vi "playlist_test.vi"() -> ()   [LabVIEW 2010]
uses:
  System.Windows.Forms
  <vilib>/Utility/miscctls.llb/LVPoint32TypeDef.ctl
  <vilib>/Utility/error.llb/DialogType.ctl
  musicplayer_glo.vi
  <vilib>/Utility/inputDevices.llb/mouseAcquire.vi
  shell32.dll
  user32.dll
panel:
  out "file count":u32
  out "drop-array":string[](array[string])
  out "win msg queue":T1
  in  "cancel":bool
  in  "ProgressBar":refnum<k24>(container)
  out "verdeckung":bool=TRUE
  in  "playlist":i32[](listbox)=[-2] caption="Playlist"
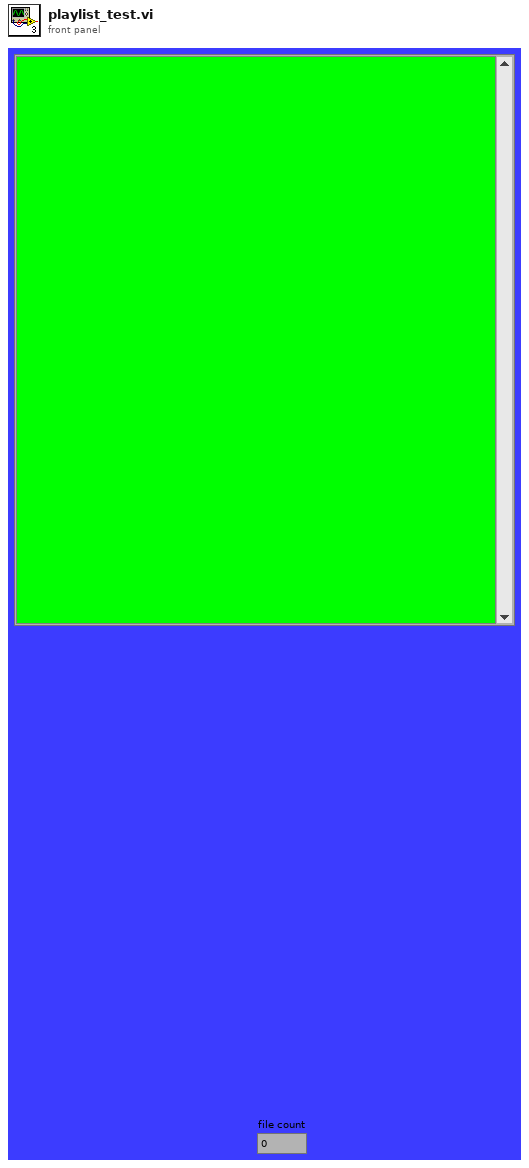
[diagram p1: front panel]
types:
  T1 = typedef "Win Msg Queue RefNum" = refnum<k1>
  T2 = enum8{"Enabled", "Disabled", "Disabled and Grayed Out"}
  T3 = enum32{"Invalid", "Standard", "Closed", "Hidden", "Minimized", "Maximized"}
  T4 = typedef "LVPoint32TypeDef.ctl" = cluster{"Horizontal":i32, "Vertical":i32}
  T5 = enum32{"Invalid", "Default", "Floating", "Floating/Auto-Hide", "Modal"}
  T6 = cluster{"Horizontal":i32, "Vertical":i32, "Scrolling":i32}
  T7 = cluster{"hWnd":u32, "Msg":u32, "wParam":u32, "lParam":i32, "time":u32, "point":cluster{"X":i32, "Y":i32}}
  T8 = typedef "DialogType.ctl" = u16
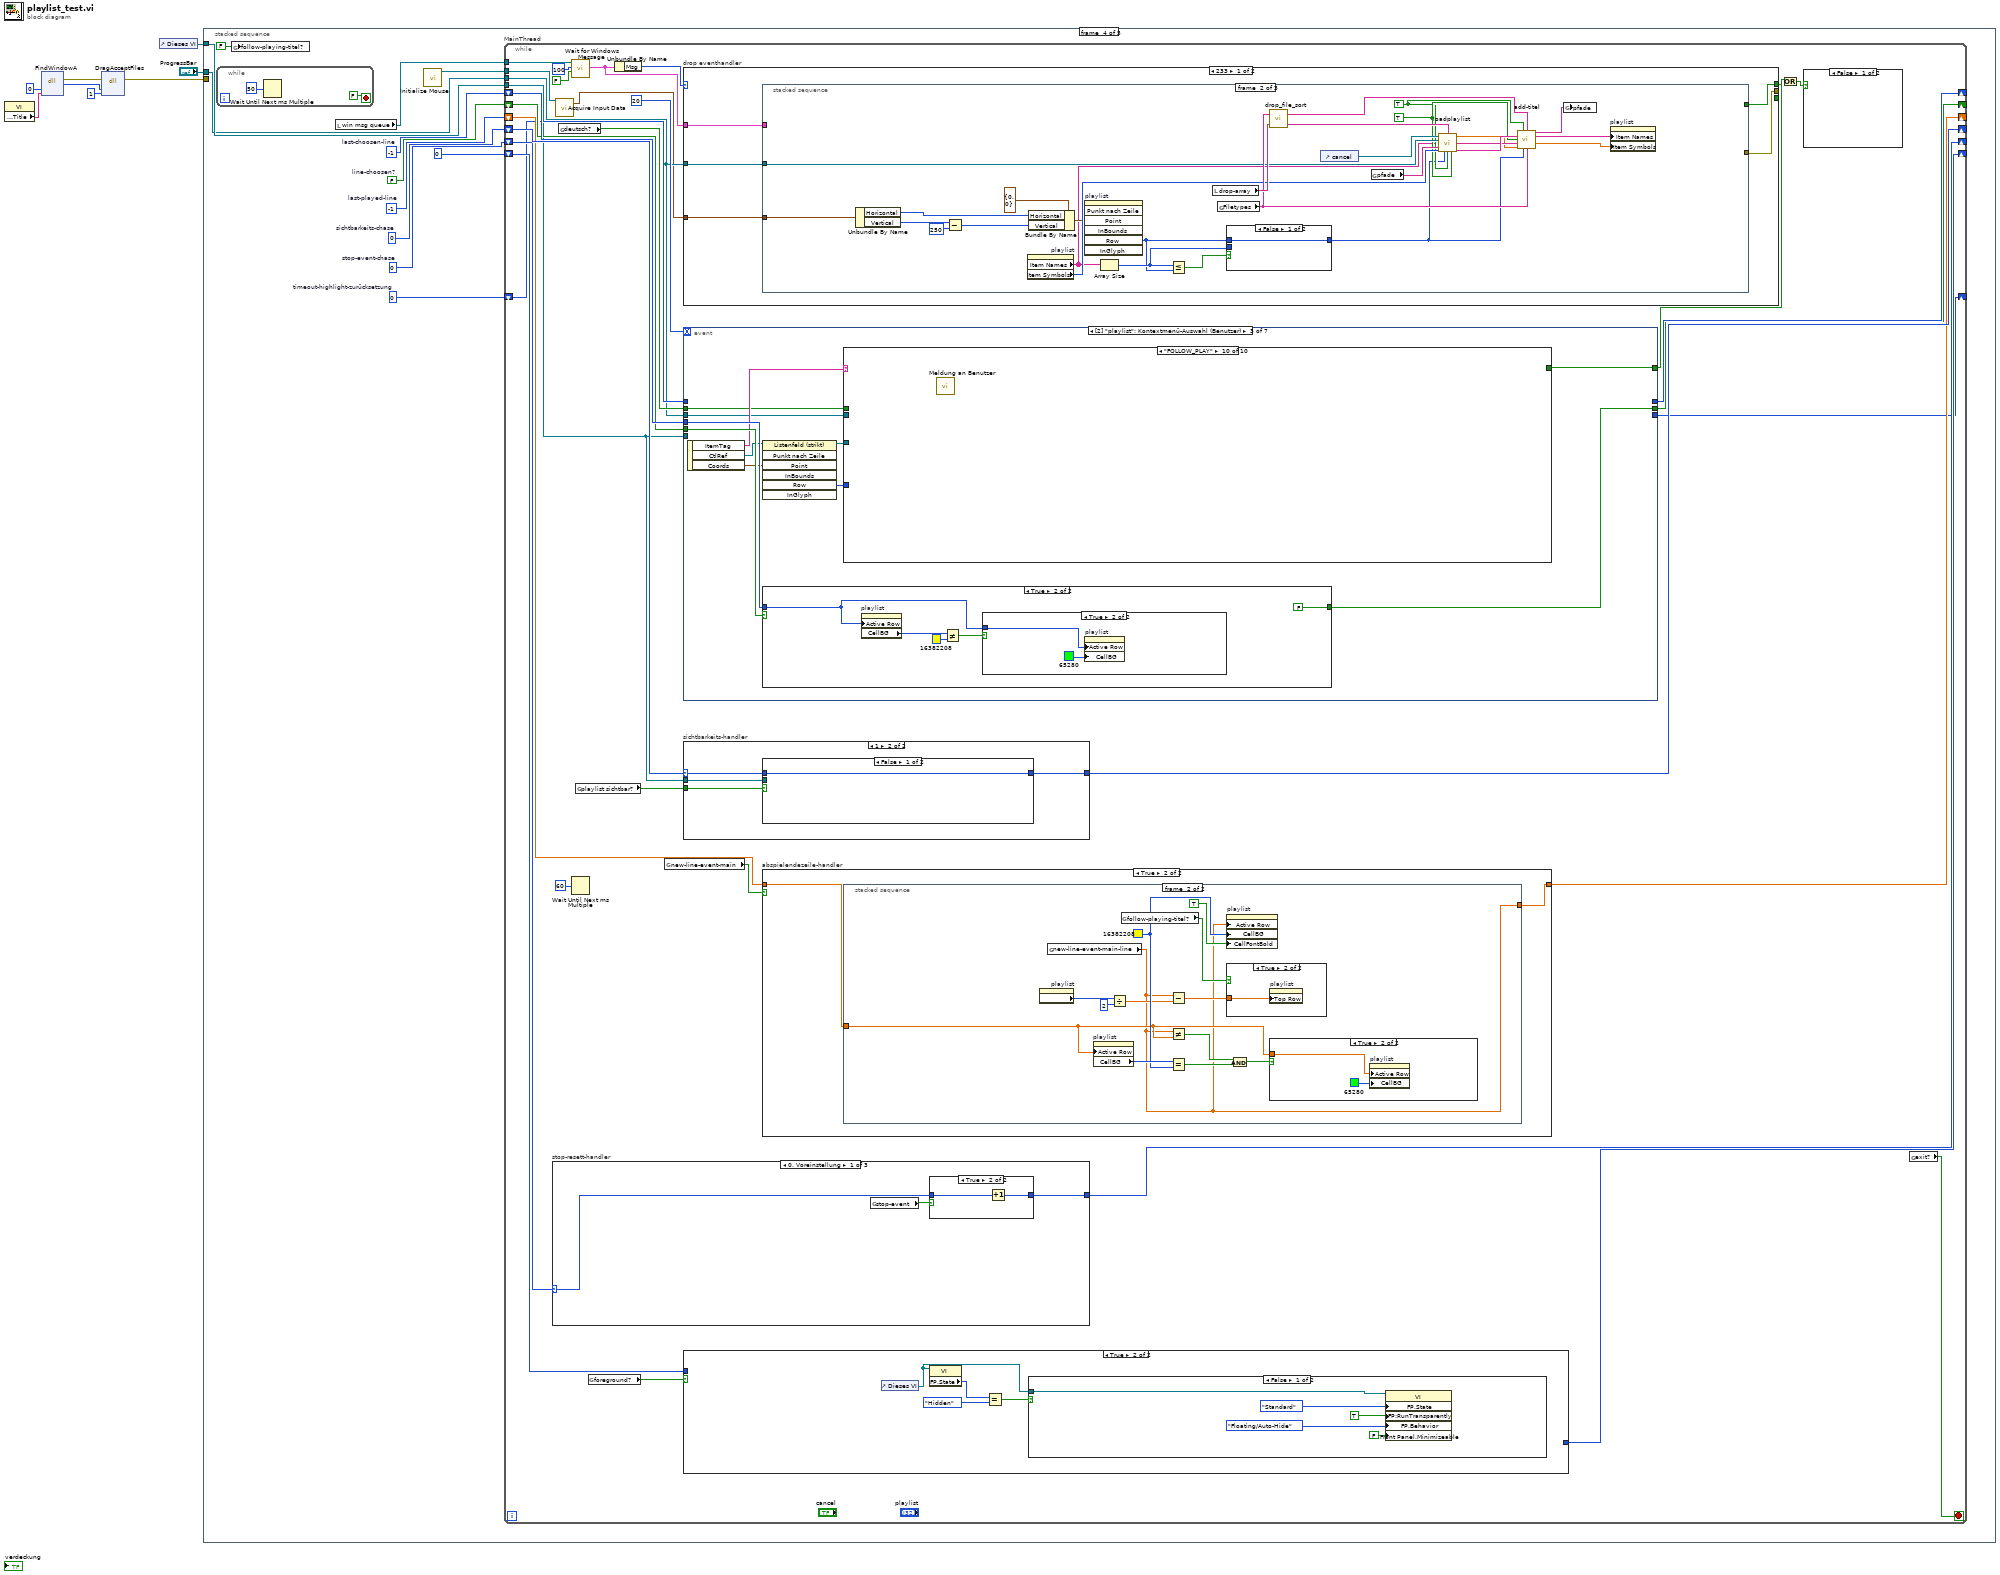
[diagram p0: block diagram]
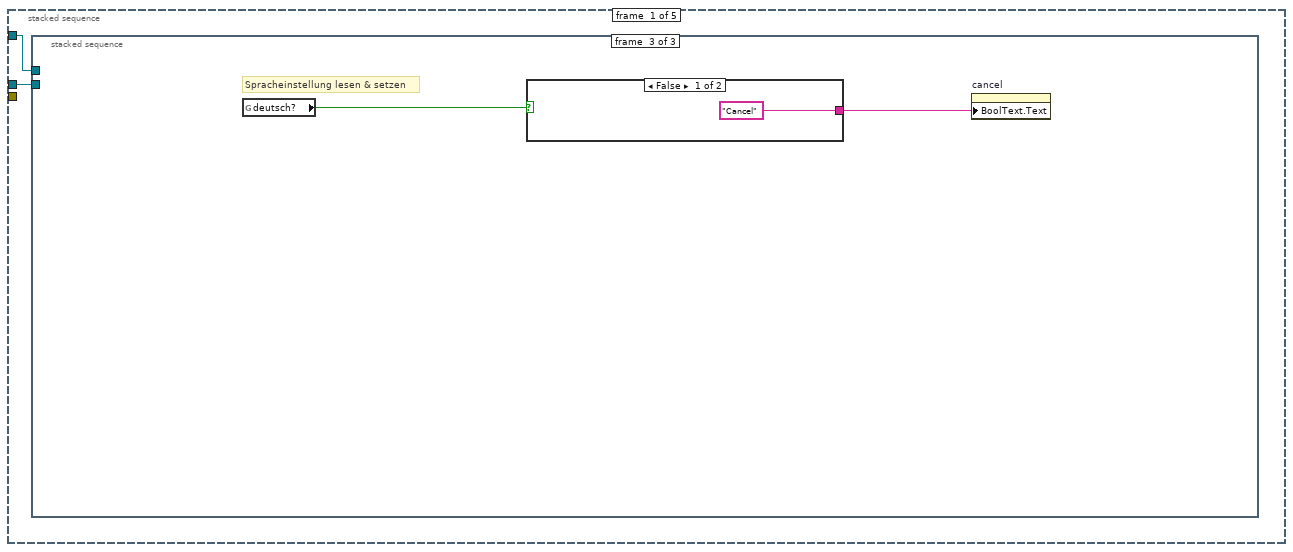
[diagram p2: hidden frame]
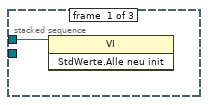
[diagram p3: hidden frame]
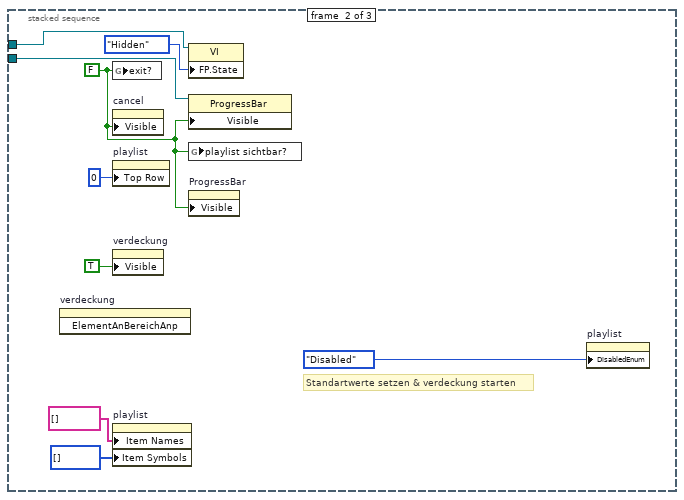
[diagram p4: hidden frame]
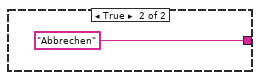
[diagram p5: hidden frame]
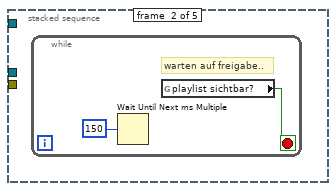
[diagram p6: hidden frame]
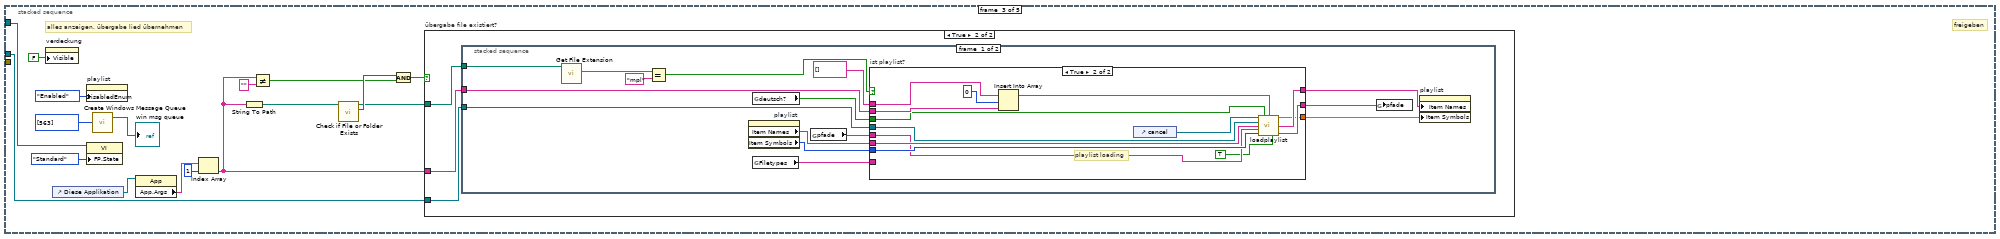
[diagram p7: hidden frame]
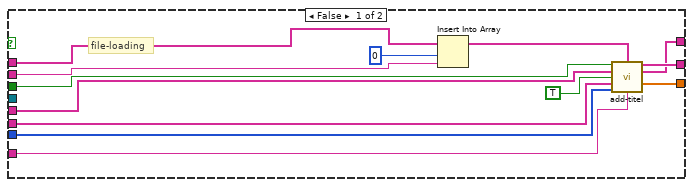
[diagram p9: hidden frame]
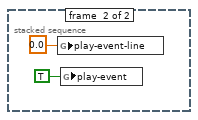
[diagram p10: hidden frame]
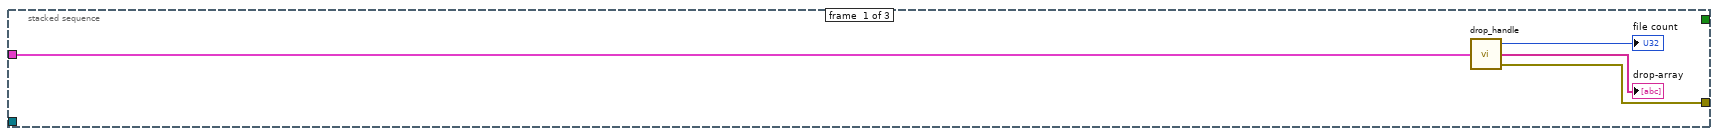
[diagram p11: hidden frame]
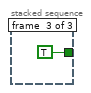
[diagram p13: hidden frame]
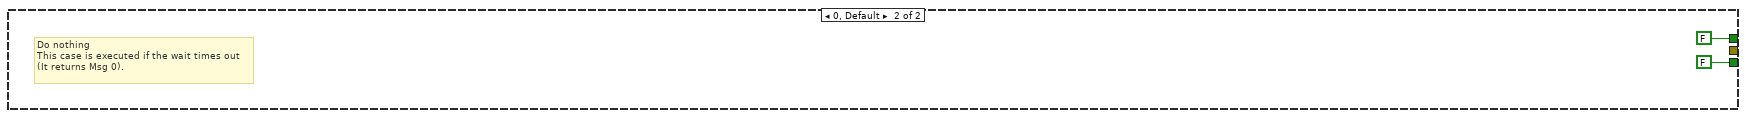
[diagram p14: hidden frame]
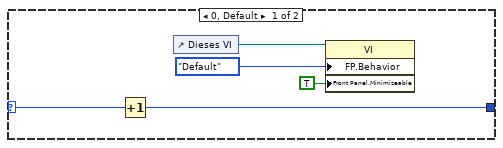
[diagram p16: hidden frame]
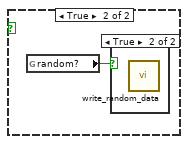
[diagram p18: hidden frame]
diagram:
  n1 = property class="VI"() -> ("Front Panel Window:Title"=w5:string)  [unwired: 2 in, 2 out]
  n2 = dll-call lib="user32.dll" fn="FindWindowA" label="FindWindow"("lpszClassName"=0, "lpszWindowName"=w5) -> (error out=w6:errorcluster, "hWnd"=w2:u32)  [unwired: 5 in, 1 out]
  n3 = dll-call lib="shell32.dll" fn="DragAcceptFiles"(error in=w6, "hWnd"=w2, "fAccept"=1) -> (error out=w1:errorcluster)  [unwired: 5 in, 1 out]
  n4 = control-ref of="Dieses VI"() -> (w8:refnum<vi>)
  n5 = stacked-sequence {
    tunnel: w8 -> [w10 _ w41 w102 w420]
    tunnel: "ProgressBar" -> [w9 _ w27 w97 _]
    tunnel: w1 -> [_ _ _ _ _]
    frame #0 {
      n6 = stacked-sequence {
        tunnel: w10 -> [w11 w17 _]
        tunnel: w9 -> [_ w13 _]
        frame #0 {
          n7 = invoke class="VI" method="StdWerte.Alle neu init"(reference=w11) -> ()  [unwired: 2 in, 3 out]
        }
        frame #1 {
          w12 = FALSE ("playlist sichtbar?")
          # "Standartwerte setzen & verdeckung starten"
          n8 = invoke on="verdeckung" class="Bool." method="ElementAnBereichAnp"() -> ()  [unwired: 3 in, 3 out]
          n9 = global write "musicplayer_glo.vi" "exit?"(w12) -> ()
          n10 = property on="cancel" class="Bool. (strikt)"("Visible"=w12) -> ()  [unwired: 2 in, 2 out]
          n11 = property on="playlist" class="Listenfeld (strikt)"("Top Row"=0 ("Erste Zeile")) -> ()  [unwired: 2 in, 2 out]
          n12 = property on="verdeckung" class="Bool."("Visible"=TRUE ("Sichtbar")) -> ()  [unwired: 2 in, 2 out]
          n13 = property on="playlist" class="Listenfeld (strikt)"("Item Names"=string[] [], "Item Symbols"=i32[] []) -> ()  [unwired: 2 in, 2 out]
          n14 = property class="VI"(reference=w17, "FP.State"=T3."Hidden" ("Frontpanel-Fenster:Status")) -> ()  [unwired: 1 in, 2 out]
          n15 = property class="ProgressBar"(reference=w13, "Visible"=w12) -> ()  [unwired: 1 in, 2 out]
          n16 = global write "musicplayer_glo.vi" "playlist sichtbar?"(w12) -> ()
          n17 = property on="ProgressBar" class="AXCont"("Visible"=w12) -> ()  [unwired: 2 in, 2 out]
          n18 = property on="playlist" class="Listenfeld (strikt)"("DisabledEnum"=T2."Disabled" ("Deaktiviert")) -> ()  [unwired: 2 in, 2 out]
        }
        frame #2 {
          # "Spracheinstellung lesen & setzen"
          n19 = global read "musicplayer_glo.vi" "deutsch?"() -> (w22:bool)
          n20 = case shown="False" w22 {
            tunnel: ["Cancel" "Abbrechen"] -> w21
            frame False {
            }
            frame True {
            }
          }
          n21 = property on="cancel" class="Bool. (strikt)"("BoolText.Text"=w21) -> ()  [unwired: 2 in, 2 out]
        }
      }
    }
    frame #1 {
      n22 = while {
        stop <- w25 stop-if-true
        # "warten auf freigabe.."
        n23 = Wait Until Next ms Multiple(millisecond multiple=u32 150 ("Vielfache von ms")) -> ()  [unwired: 1 out]
        n24 = global read "musicplayer_glo.vi" "playlist sichtbar?"() -> (w25:bool)
      }
    }
    frame #2 {
      # "alles anzeigen, übergabe lied übernehmen"
      # "freigeben"
      n25 = property on="verdeckung" class="Bool."("Visible"=FALSE ("Sichtbar")) -> ()  [unwired: 2 in, 2 out]
      n26 = control-ref of="Diese Applikation"() -> (w37:refnum<vi>)
      n27 = property on="playlist" class="Listenfeld (strikt)"("DisabledEnum"=T2."Enabled" ("Deaktiviert")) -> ()  [unwired: 2 in, 2 out]
      n28 = property class="VI"(reference=w41, "FP.State"=T3."Standard" ("Frontpanel-Fenster:Status")) -> ()  [unwired: 1 in, 2 out]
      n29 = call <userlib>:"Create Windows Message Queue.vi"("Messeges (none)"=u32[] [563]) -> ("win msg queue"=→"win msg queue":T1)  [unwired: 2 in, 1 out]
      n30 = property class="App"(reference=w37) -> ("App.Args"=w36:string[])  [unwired: 1 in, 2 out]
      n31 = Index Array(array=w36, index=1 ("Index")) -> (element=w31:string)
      n32 = String To Path(string=w31) -> (path=w34:path)
      n33 = Not Equal?(x=w31, y="") -> (x != y?=w28:bool)
      n34 = call <vilib>:"Check if File or Folder Exists.vi"("path"=w34) -> ("file or folder exists?"=w33:bool, "dup path"=w32:path)  [unwired: 8 in, 1 out]
      n35 = And(x=w33, y=w28) -> (x .and. y?=w29:bool)
      n36 = case "übergabe file existiert?" shown="True" w29 {
        tunnel: w32 -> [_ w46]
        tunnel: w31 -> [_ w45]
        tunnel: w27 -> [_ w44]
        frame False {
        }
        frame True {
          n37 = stacked-sequence {
            tunnel: w46 -> [w61 _]
            tunnel: w45 -> [w53 _]
            tunnel: w44 -> [w47 _]
            frame #0 {
              n38 = call <vilib>:"Get File Extension.vi"("file"=w61) -> ("lowercase file extension"=w60:string)  [unwired: 7 in, 3 out]
              n39 = Equal?(x=w60, y="mpl") -> (x = y?=w58:bool)
              n40 = property on="playlist" class="Listenfeld (strikt)"() -> ("Item Names"=w55:string[], "Item Symbols"=w54:i32[])  [unwired: 2 in, 2 out]
              n41 = global read "musicplayer_glo.vi" "deutsch?"() -> (w57:bool)
              n42 = global read "musicplayer_glo.vi" "Filetypes"() -> (w52:string)
              n43 = global read "musicplayer_glo.vi" "pfade"() -> (w56:string[])
              n44 = case "ist playlist?" shown="True" w58 {
                tunnel: w57 -> [w74 w84]
                tunnel: w56 -> [w73 w81]
                tunnel: w55 -> [w71 w83]
                tunnel: w54 -> [w70 w82]
                tunnel: w53 -> [w68 w86]
                tunnel: w52 -> [w66 _]
                tunnel: [w65 w79] -> w51
                tunnel: [w64 w78] -> w50
                tunnel: [w63 w77] -> w49
                tunnel: string[] [] -> [w62 w87]
                tunnel: w47 -> [_ w76]
                frame False {
                  # "file-loading"
                  n45 = Insert Into Array(array=w62, index=0 ("Index"), new element=w68) -> (w67:string[])
                  n46 = call "add-titel.vi"("deutsch?"=w74, "input-array"=w67, "pfade"=w73, "use input-array?"=TRUE, "playlist"=w71, "symbole"=w70, "dateitypen"=w66) -> ("pfade out"=w65:string[], "playlist out"=w64:string[], "symbole out"=w63:dbl[])  [unwired: 6 in]
                }
                frame True {
                  # "playlist loading"
                  n47 = Insert Into Array(array=w87, index=0 ("Index"), new element=w86) -> (w85:string[])
                  n48 = control-ref of="cancel"() -> (w75:refnum<vi>)
                  n49 = call "loadplaylist.vi"("Boolesch-ref"=w75, "deutsch?"=w84, "input-array"=w85, "ProgressBar-ref"=w76, "playlist-input"=w83, "pfade-in"=w81, "symbole-in"=w82, "von input-array?"=TRUE) -> ("symbole-out"=w77:dbl[], "playlist-output"=w78:string[], "pfade-out"=w79:string[])  [unwired: 5 in]
                }
              }
              n50 = global write "musicplayer_glo.vi" "pfade"(w51) -> ()
              n51 = property on="playlist" class="Listenfeld (strikt)"("Item Names"=w50, "Item Symbols"=w49) -> ()  [unwired: 2 in, 2 out]
            }
            frame #1 {
              n52 = global write "musicplayer_glo.vi" "play-event-line"(0.0 ("play-event-line")) -> ()
              n53 = global write "musicplayer_glo.vi" "play-event"(TRUE ("play-event-playlist")) -> ()
            }
          }
        }
      }
    }
    frame #3 {
      w94 = 0  # timeout-highlight-zurücksetzung
      w96 = 0  # stop-event-chase
      w98 = -1  # last-played-line
      w99 = FALSE  # line-choosen?
      w100 = -1  # last-choosen-line
      w101 = 0  # sichtbarkeits-chase
      n54 = while {
        stop <- FALSE stop-if-true
        n55 = Wait Until Next ms Multiple(millisecond multiple=u32 50 ("Vielfache von ms")) -> ()  [unwired: 1 out]
      }
      n56 = global write "musicplayer_glo.vi" "follow-playing-titel?"(FALSE ("follow-playing-titel?")) -> ()
      n57 = local read "win msg queue"() -> (w93:T1)
      n58 = call <vilib>:"Initialize Mouse.vi"() -> ("device ID"=w92:refnum<k1>)  [unwired: 10 in, 1 out]
      n59 = while "MainThread" {
        tunnel: w102 -> [w108]
        shift-right: [w134] -> _
        shift-left: w101 -> [w136]
        shift-right: [w129] -> _
        shift-left: w99 -> [w131]
        shift-right: [w130] -> _
        shift-left: w100 -> [w132]
        shift-right: [w126] -> _
        shift-left: w98 -> [w127]
        tunnel: w97 -> [w107]
        shift-right: [w123] -> _
        shift-left: w96 -> [w124]
        shift-right: [w119] -> _
        shift-left: 0 -> [w118]
        shift-right: [w116] -> _
        shift-left: w94 -> [w117]
        tunnel: w93 -> [w114]
        tunnel: w92 -> [w106]
        stop <- w122 stop-if-true
        n60 = case "stop-resett-handler" shown="0, Voreinstellung" w124 {
          selector: w124 -> [w199 w205 w216]
          tunnel: [w198 w204 w215] -> w123
          frame 0, Default {
            n61 = global read "musicplayer_glo.vi" "stop-event"() -> (w200:bool)
            n62 = case shown="True" w200 {
              tunnel: w199 -> [w201 w203]
              tunnel: [w201 w202] -> w198
              frame False {
              }
              frame True {
                n63 = Increment(x=w203) -> (x+1=w202:i32)
              }
            }
          }
          frame 1 {
            n64 = property on="playlist" class="Listenfeld (strikt)"() -> ("Item Names"=w208:string[])  [unwired: 2 in, 2 out]
            n65 = Array Size(array=w208) -> (size(s)=w207:i32)
            n66 = for {
              N: w207 -> [_]
              i -> [w213]
              n67 = property on="playlist" class="Listenfeld (strikt)"("Active Row"=w213, "CellFontBold"=FALSE ("Aktive Zeile:Schriftart der Zelle:Fett"), "CellBG"=u32 65280 ("Farbfeld 2")) -> ()  [unwired: 2 in, 2 out]
            }
            n68 = global read "musicplayer_glo.vi" "stop-event"() -> (w206:bool)
            n69 = case shown="True" w206 {
              tunnel: [0 w210] -> w204
              tunnel: w205 -> [_ w211]
              frame False {
              }
              frame True {
                n70 = Increment(x=w211) -> (x+1=w210:i32)
              }
            }
          }
          frame 2 {
            n71 = global read "musicplayer_glo.vi" "stop-event"() -> (w217:bool)
            n72 = case shown="True" w217 {
              tunnel: [0 w219] -> w215
              tunnel: w216 -> [_ w219]
              frame False {
              }
              frame True {
              }
            }
          }
        }
        n73 = call-poly <vilib>:"Acquire Input Data.vi"("device ID"=w106) -> ("axis info"=w105:T6)  [unwired: 15 in, 3 out]
        n74 = global read "musicplayer_glo.vi" "deutsch?"() -> (w125:bool)
        n75 = call <userlib>:"Wait for Windows Message.vi"("win msg queue"=w114, "ms timeout (-1)"=100, "ignore previous (F)"=FALSE ("ignore previous (T)")) -> ("Message"=w109:T7)  [unwired: 1 in, 5 out]
        n76 = Wait Until Next ms Multiple(millisecond multiple=u32 60 ("Vielfache von ms")) -> ()  [unwired: 1 out]
        n77 = global read "musicplayer_glo.vi" "playlist sichtbar?"() -> (w135:bool)
        n78 = global read "musicplayer_glo.vi" "foreground?"() -> (w120:bool)
        n79 = Unbundle By Name(w109) -> ("Msg"=w112:u32)
        n80 = global read "musicplayer_glo.vi" "new-line-event-main"() -> (w128:bool)
        n81 = case "drop eventhandler" shown="233" w112 {
          tunnel: [_ FALSE] -> _
          tunnel: [w140 _] -> _
          tunnel: [w141 FALSE] -> w110
          tunnel: w109 -> [w142 _]
          tunnel: w107 -> [w139 _]
          tunnel: w105 -> [w138 _]
          frame 563 {
            n82 = stacked-sequence {
              tunnel: [w146 _ _] -> w140
              tunnel: w142 -> [w145 _ _]
              tunnel: [_ _ TRUE] -> w141
              tunnel: w139 -> [_ w167 _]
              tunnel: w138 -> [_ w156 _]
              frame #0 {
                n83 = call "drop_handle.vi"("Message"=w145) -> ("error out"=w146:errorcluster, "drop-array"=→"drop-array":string[], "file count"=→"file count":u32)
              }
              frame #1 {
                w152 = TRUE ("ab position?")
                w160 = TRUE ("use input-array?")
                n84 = Unbundle By Name(w156) -> ("Horizontal"=w159:i32, "Vertical"=w155:i32)
                n85 = Subtract(x=w155, y=250) -> (x-y=w154:i32)
                n86 = property on="playlist" class="Listenfeld (strikt)"() -> ("Item Names"=w151:string[], "Item Symbols"=w162:i32[])  [unwired: 2 in, 2 out]
                n87 = Bundle By Name(cluster=T4 {"Horizontal"=0, "Vertical"=0} ("Koordinaten"), "Horizontal"=w159, "Vertical"=w154) -> (w157:T4)
                n88 = invoke on="playlist" class="Listenfeld (strikt)" method="Punkt nach Zeile"("Point"=w157) -> ("Row"=w147:i32)  [unwired: 6 in, 6 out]
                n89 = Array Size(array=w151) -> (size(s)=w150:i32)
                n90 = Less Or Equal?(x=w150, y=w147) -> (x <= y?=w149:bool)
                n91 = local read "drop-array"() -> (w174:string[])
                n92 = global read "musicplayer_glo.vi" "Filetypes"() -> (w170:string)
                n93 = case shown="False" w149 {
                  tunnel: w150 -> [_ w176]
                  tunnel: [w175 w176] -> w148
                  tunnel: w147 -> [w175 _]
                  frame False {
                  }
                  frame True {
                  }
                }
                n94 = call "drop_file_sort.vi"("drop-array"=w174, "filetypes"=w170) -> ("playlist-array"=w161:string[], "file-array"=w169:string[])
                n95 = control-ref of="cancel"() -> (w168:refnum<vi>)
                n96 = global read "musicplayer_glo.vi" "pfade"() -> (w166:string[])
                n97 = call "loadplaylist.vi"("Boolesch-ref"=w168, "input-array"=w161, "ProgressBar-ref"=w167, "playlist-input"=w151, "pfade-in"=w166, "symbole-in"=w162, "ab position"=w148, "ab position?"=w152, "von input-array?"=w160) -> ("symbole-out"=w163:dbl[], "playlist-output"=w164:string[], "pfade-out"=w165:string[])  [unwired: 4 in]
                n98 = call "add-titel.vi"("abposeinfügen"=w152, "input-array"=w169, "pfade"=w165, "use input-array?"=w160, "playlist"=w164, "symbole"=w163, "pos"=w148, "dateitypen"=w170) -> ("pfade out"=w173:string[], "playlist out"=w172:string[], "symbole out"=w171:dbl[])  [unwired: 5 in]
                n99 = global write "musicplayer_glo.vi" "pfade"(w173) -> ()
                n100 = property on="playlist" class="Listenfeld (strikt)"("Item Names"=w172, "Item Symbols"=w171) -> ()  [unwired: 2 in, 2 out]
              }
              frame #2 {
              }
            }
          }
          frame 0, Default {
            # "Do nothing\nThis case is executed if the wait times out\n(It returns Msg 0)."
          }
        }
        n101 = event "Ereignisstruktur" shown="[2] \"playlist\": Kontextmenü-Auswahl (Benutzer)" {
          selector: _ -> [_ _ _ _ _ _ _]
          dyn-events: _ -> [_ _ _ _ _ _ _]
          timeout: 20 -> [_ _ _ _ _ _ _]
          tunnel: w108 -> [_ _ _ _ _ _ _]
          tunnel: w132 -> [_ _ w305 _ w400 w412 w417]
          tunnel: w131 -> [_ _ w304 _ w401 w411 w416]
          tunnel: [_ w273 _ _ _ w412 w417] -> w130
          tunnel: [_ TRUE w303 _ w399 w411 w416] -> w129
          tunnel: [_ _ w301 _ _ _ _] -> w121
          tunnel: w107 -> [_ _ w300 _ _ _ _]
          tunnel: w125 -> [_ _ w295 _ _ _ _]
          tunnel: w117 -> [_ _ _ _ _ w410 _]
          tunnel: [_ _ _ _ _ w409 _] -> w116
          event "playlist": Double Click {
            n102 = event-data() -> ("Coords"=w259:T4, "CtlRef"=w260:refnum<vi>)  [unwired: 1 in]
            n103 = invoke class="Listenfeld (strikt)" method="Punkt nach Zeile"(reference=w260, "Point"=w259) -> ("Row"=w258:i32)  [unwired: 5 in, 6 out]
            n104 = global read "musicplayer_glo.vi" "pfade"() -> (w263:string[])
            n105 = Index Array(array=w263, index=w258) -> (element=w261:string)
            n106 = Not Equal?(x=w261, y="") -> (x != y?=w257:bool)
            n107 = case shown="True" w257 {
              tunnel: w260 -> [_ w265]
              tunnel: w258 -> [_ w264]
              frame False {
              }
              frame True {
                n108 = stacked-sequence {
                  tunnel: w265 -> [_ _]
                  tunnel: w264 -> [w267 _]
                  frame #0 {
                    n109 = global write "musicplayer_glo.vi" "play-event-line"(w267) -> ()
                    n110 = property on="playlist" class="Listenfeld (strikt)"() -> ("Item Symbols"=w269:i32[])  [unwired: 2 in, 2 out]
                    n111 = Replace Array Subset(array=w269, new element=38, index=w267) -> (w268:i32[])
                    n112 = property on="playlist" class="Listenfeld (strikt)"("Item Symbols"=w268) -> ()  [unwired: 2 in, 2 out]
                  }
                  frame #1 {
                    n113 = global write "musicplayer_glo.vi" "play-event"(TRUE ("play-event-playlist")) -> ()
                  }
                }
              }
            }
          }
          event "playlist": Shortcut Menu Activation? {
            w282 = T8 0 items=["no dialog", "OK message", "continue or stop message", "OK message + warnings", "continue/stop + warnings"] ("type of dialog (OK msg:1)")
            n114 = event-data() -> ("MenuRef"=w291:refnum<k9>, "Coords"=w289:T4, "CtlRef"=w287:refnum<vi>)  [unwired: 1 in]
            n115 = invoke class="Listenfeld (strikt)" method="Punkt nach Zeile"(reference=w287, "Point"=w289) -> (reference out=w276:refnum<vi>, "Row"=w273:i32)  [unwired: 5 in, 5 out]
            n116 = property class="Listenfeld (strikt)"(reference=w287) -> ("Item Names"=w288:string[])  [unwired: 1 in, 2 out]
            n117 = property class="Listenfeld (strikt)"(reference=w276, "Active Row"=w273) -> (reference out=w275:refnum<vi>, "CellBG"=w274:u32)  [unwired: 1 in, 1 out]
            n118 = Index Array(array=w288, index=w273) -> (element=w286:string)
            n119 = global read "musicplayer_glo.vi" "follow-playing-titel?"() -> (w277:bool)
            n120 = Not Equal?(x=w286, y="") -> (x != y?=w284:bool)
            n121 = Not Equal?(x=w274, y=u32 16382208 ("Farbfeld 2")) -> (x != y?=w272:bool)
            n122 = case shown="True" w272 {
              tunnel: w275 -> [_ w293]
              tunnel: w273 -> [_ w292]
              frame False {
              }
              frame True {
                n123 = property class="Listenfeld (strikt)"(reference=w293, "Active Row"=w292, "CellBG"=u32 13816530 ("Farbfeld 2")) -> ()  [unwired: 1 in, 2 out]
              }
            }
            n124 = Set Menu Item Info(7:"REMOVE_TITEL" ("Menüpunkt-Tag"), 9:w284, 11:w291) -> (0:w279:errorcluster, 3:w280:refnum<k9>)  [unwired: 2 in, 2 out]
            n125 = Set Menu Item Info(6:w277, 7:"FOLLOW_PLAY", 8:w279, 11:w280) -> (0:w278:errorcluster)  [unwired: 2 in, 2 out]
            n126 = call <vilib>:"Simple Error Handler.vi"("type of dialog (OK msg:1)"=w282, "error in (no error)"=w278) -> ()  [unwired: 1 in, 7 out]
            n127 = event-data() -> ()  [unwired: 2 in, 1 out]
          }
          event "playlist": Shortcut Menu Selection (User) {
            n128 = event-data() -> ("ItemTag"=w302:string, "CtlRef"=w297:refnum<vi>, "Coords"=w299:T4)  [unwired: 1 in]
            n129 = invoke class="Listenfeld (strikt)" method="Punkt nach Zeile"(reference=w297, "Point"=w299) -> (reference out=w296:refnum<vi>, "Row"=w298:i32)  [unwired: 5 in, 5 out]
            n130 = case shown="True" w304 {
              tunnel: w305 -> [_ w383]
              tunnel: [_ FALSE] -> w303
              frame False {
              }
              frame True {
                n131 = property on="playlist" class="Listenfeld (strikt)"("Active Row"=w383) -> ("CellBG"=w385:u32)  [unwired: 2 in, 2 out]
                n132 = Not Equal?(x=w385, y=u32 16382208 ("Farbfeld 2")) -> (x != y?=w384:bool)
                n133 = case shown="True" w384 {
                  tunnel: w383 -> [_ w387]
                  frame False {
                  }
                  frame True {
                    n134 = property on="playlist" class="Listenfeld (strikt)"("Active Row"=w387, "CellBG"=u32 65280 ("Farbfeld 2")) -> ()  [unwired: 2 in, 2 out]
                  }
                }
              }
            }
            n135 = case shown="\"FOLLOW_PLAY\"" w302 {
              tunnel: [FALSE TRUE _ _ TRUE TRUE _ TRUE TRUE _] -> w301
              tunnel: w300 -> [_ w310 _ _ _ _ _ _ _ _]
              tunnel: w298 -> [_ w309 _ w335 _ w349 _ w361 _ _]
              tunnel: w296 -> [_ _ _ _ _ _ _ _ _ _]
              tunnel: w295 -> [_ w308 w330 _ _ w357 _ _ _ _]
              frame "default", Default {
              }
              frame "LOAD_PLAYLIST" {
                n136 = stacked-sequence {
                  tunnel: w310 -> [w313 w320 w329]
                  tunnel: w309 -> [_ w316 _]
                  tunnel: w308 -> [_ _ _]
                  frame #0 {
                    w311 = TRUE ("Sichtbar")
                    # "show cancel & statbar"
                    n137 = property on="ProgressBar" class="AXCont"("Visible"=w311) -> ()  [unwired: 2 in, 2 out]
                    n138 = property on="cancel" class="Bool. (strikt)"("Visible"=w311) -> ()  [unwired: 2 in, 2 out]
                    n139 = property on="verdeckung" class="Bool."("Visible"=w311) -> ()  [unwired: 2 in, 2 out]
                    n140 = property class="ProgressBar"(reference=w313, "Visible"=w311, "Value"=0) -> ()  [unwired: 1 in, 2 out]
                  }
                  frame #1 {
                    # "load playlist via subvi"
                    n141 = global read "musicplayer_glo.vi" "pfade"() -> (w327:string[])
                    n142 = Index Array(array=w327, index=w316) -> (element=w326:string)
                    n143 = global read "musicplayer_glo.vi" "deutsch?"() -> (w319:bool)
                    n144 = property on="playlist" class="Listenfeld (strikt)"() -> ("Item Names"=w321:string[], "Item Symbols"=w322:i32[])  [unwired: 2 in, 2 out]
                    n145 = control-ref of="cancel"() -> (w324:refnum<vi>)
                    n146 = Not Equal?(x=w326, y="") -> (x != y?=w317:bool)
                    n147 = global read "musicplayer_glo.vi" "pfade"() -> (w323:string[])
                    n148 = call "loadplaylist.vi"("Boolesch-ref"=w324, "deutsch?"=w319, "ProgressBar-ref"=w320, "playlist-input"=w321, "pfade-in"=w323, "symbole-in"=w322, "ab position"=w316, "ab position?"=w317) -> ("symbole-out"=w318:dbl[], "playlist-output"=w314:string[], "pfade-out"=w315:string[])  [unwired: 5 in]
                    n149 = global write "musicplayer_glo.vi" "pfade"(w315) -> ()
                    n150 = property on="playlist" class="Listenfeld (strikt)"("Item Names"=w314, "Item Symbols"=w318) -> ()  [unwired: 2 in, 2 out]
                  }
                  frame #2 {
                    w328 = FALSE
                    n151 = property on="cancel" class="Bool. (strikt)"("Visible"=w328) -> ()  [unwired: 2 in, 2 out]
                    n152 = property class="ProgressBar"(reference=w329, "Visible"=w328) -> ()  [unwired: 1 in, 2 out]
                    n153 = property on="ProgressBar" class="AXCont"("Visible"=w328) -> ()  [unwired: 2 in, 2 out]
                    n154 = property on="verdeckung" class="Bool."("Visible"=w328) -> ()  [unwired: 2 in, 2 out]
                  }
                }
              }
              frame "SAVE_PLAYLIST" {
                n155 = global read "musicplayer_glo.vi" "pfade"() -> (w331:string[])
                n156 = call "saveplaylist.vi"("pfade"=w331, "deutsch?"=w330) -> ()  [unwired: 10 in]
              }
              frame "PLAY_TITEL" {
                n157 = global read "musicplayer_glo.vi" "pfade"() -> (w336:string[])
                n158 = Index Array(array=w336, index=w335) -> (element=w334:string)
                n159 = Not Equal?(x="" ("Element"), y=w334) -> (x != y?=w332:bool)
                n160 = case shown="True" w332 {
                  tunnel: w335 -> [_ w337]
                  frame False {
                  }
                  frame True {
                    n161 = stacked-sequence {
                      tunnel: w337 -> [w338 _]
                      frame #0 {
                        n162 = global write "musicplayer_glo.vi" "play-event-line"(w338) -> ()
                      }
                      frame #1 {
                        n163 = global write "musicplayer_glo.vi" "play-event"(TRUE ("play-event-playlist")) -> ()
                      }
                    }
                  }
                }
              }
              frame "CLEAR_PLAYLIST" {
                n164 = stacked-sequence {
                  frame #0 {
                    w342 = string[] [] ("pfade")
                    n165 = global write "musicplayer_glo.vi" "pfade"(w342) -> ()
                    n166 = property on="playlist" class="Listenfeld (strikt)"("Item Names"=w342, "Item Symbols"=i32[] [] ("Objektsymbole")) -> ()  [unwired: 2 in, 2 out]
                  }
                  frame #1 {
                    n167 = property on="playlist" class="Listenfeld (strikt)"("Top Row"=0 ("Erste Zeile")) -> ()  [unwired: 2 in, 2 out]
                  }
                }
              }
              frame "ADD_TITEL" {
                n168 = global read "musicplayer_glo.vi" "pfade"() -> (w351:string[])
                n169 = Index Array(array=w351, index=w349) -> (element=w353:string)
                n170 = property on="playlist" class="Listenfeld (strikt)"() -> ("Item Names"=w354:string[], "Item Symbols"=w345:i32[])  [unwired: 2 in, 2 out]
                n171 = global read "musicplayer_glo.vi" "Filetypes"() -> (w348:string)
                n172 = Not Equal?(x=w353, y="") -> (x != y?=w350:bool)
                n173 = call "add-titel.vi"("deutsch?"=w357, "abposeinfügen"=w350, "pfade"=w351, "use input-array?"=FALSE, "playlist"=w354, "symbole"=w345, "pos"=w349, "dateitypen"=w348) -> ("pfade out"=w356:string[], "playlist out"=w355:string[], "symbole out"=w344:dbl[])  [unwired: 5 in]
                n174 = global write "musicplayer_glo.vi" "pfade"(w356) -> ()
                n175 = property on="playlist" class="Listenfeld (strikt)"("Item Names"=w355, "Item Symbols"=w344) -> ()  [unwired: 2 in, 2 out]
              }
              frame "Tick all" {
                n176 = global read "musicplayer_glo.vi" "pfade"() -> (w359:string[])
                n177 = call "tickall.vi"("pfade"=w359) -> ("symbole out"=w358:dbl[])  [unwired: 10 in]
                n178 = property on="playlist" class="Listenfeld (strikt)"("Item Symbols"=w358) -> ()  [unwired: 2 in, 2 out]
              }
              frame "REMOVE_TITEL" {
                n179 = global read "musicplayer_glo.vi" "pfade"() -> (w363:string[])
                n180 = Index Array(array=w363, index=w361) -> (element=w365:string)
                n181 = Not Equal?(x=w365, y="") -> (x != y?=w362:bool)
                n182 = case shown="True" w362 {
                  tunnel: w363 -> [_ w372]
                  tunnel: w361 -> [_ w370]
                  frame False {
                  }
                  frame True {
                    n183 = property on="playlist" class="Listenfeld (strikt)"() -> ("Item Names"=w367:string[], "Item Symbols"=w366:i32[])  [unwired: 2 in, 2 out]
                    n184 = call "deletetitel.vi"("pos"=w370, "symbole"=w366, "playlist"=w367, "pfade"=w372) -> ("symbole out"=w369:dbl[], "playlist out"=w368:string[], "pfade out"=w371:string[])  [unwired: 5 in]
                    n185 = global write "musicplayer_glo.vi" "pfade"(w371) -> ()
                    n186 = property on="playlist" class="Listenfeld (strikt)"("Item Names"=w368, "Item Symbols"=w369) -> ()  [unwired: 2 in, 2 out]
                  }
                }
              }
              frame "REMOVE_NOT_AKTIVATED" {
                n187 = stacked-sequence {
                  frame #0 {
                    n188 = property on="playlist" class="Listenfeld (strikt)"() -> ("Item Names"=w376:string[], "Item Symbols"=w375:i32[])  [unwired: 2 in, 2 out]
                    n189 = global read "musicplayer_glo.vi" "pfade"() -> (w374:string[])
                    n190 = call "removenotticket.vi"("symbole"=w375, "playlist"=w376, "pfade"=w374) -> ("symbole out"=w379:dbl[], "playlist out"=w378:string[], "pfade out"=w377:string[])  [unwired: 6 in]
                    n191 = global write "musicplayer_glo.vi" "pfade"(w377) -> ()
                    n192 = property on="playlist" class="Listenfeld (strikt)"("Item Names"=w378, "Item Symbols"=w379) -> ()  [unwired: 2 in, 2 out]
                  }
                  frame #1 {
                    n193 = property on="playlist" class="Listenfeld (strikt)"("Top Row"=0 ("Erste Zeile")) -> ()  [unwired: 2 in, 2 out]
                  }
                }
              }
              frame "FOLLOW_PLAY" {
                n194 = call "Meldung an Benutzer"() -> ()  [unwired: 10 in, 2 out]
              }
            }
          }
          event "playlist": Value Change {
            n195 = event-data() -> ("NewVal"=w388:i32[])  [unwired: 1 in]
            n196 = Array Size(array=w388) -> (size(s)=w389:i32)
            n197 = for {
              N: w389 -> [_]
              tunnel: w388 -> [w390]
              w396 = 37
              n198 = property on="playlist" class="Listenfeld (strikt)"() -> ("Item Symbols"=w397:i32[])  [unwired: 2 in, 2 out]
              n199 = Index Array(array=w390) -> (element=w392:i32)  [unwired: 1 in]
              n200 = Index Array(array=w397, index=w392) -> (element=w394:i32)
              n201 = Equal?(x=w394, y=w396) -> (x = y?=w393:bool)
              n202 = Select(t=38, s=w393, f=w396) -> (s? t:f=w398:i32)
              n203 = Replace Array Subset(array=w397, new element=w398, index=w392) -> (w391:i32[])
              n204 = property on="playlist" class="Listenfeld (strikt)"("Item Symbols"=w391) -> ()  [unwired: 2 in, 2 out]
            }
          }
          event Mouse Down {
            n205 = event-data() -> ()  [unwired: 1 in, 3 out]
            n206 = case shown="False" w401 {
              tunnel: w400 -> [_ w404]
              tunnel: [_ FALSE] -> w399
              frame False {
              }
              frame True {
                n207 = property on="playlist" class="Listenfeld (strikt)"("Active Row"=w404) -> ("CellBG"=w406:u32)  [unwired: 2 in, 2 out]
                n208 = Not Equal?(x=w406, y=u32 16382208 ("Farbfeld 2")) -> (x != y?=w405:bool)
                n209 = case shown="True" w405 {
                  tunnel: w404 -> [_ w408]
                  frame False {
                  }
                  frame True {
                    n210 = property on="playlist" class="Listenfeld (strikt)"("Active Row"=w408, "CellBG"=u32 65280 ("Farbfeld 2")) -> ()  [unwired: 2 in, 2 out]
                  }
                }
              }
            }
          }
          event Timeout {
            n211 = event-data() -> ()  [unwired: 1 in, 2 out]
            n212 = case shown="1" w410 {
              selector: w410 -> [_ w415]
              tunnel: [1 w415] -> w409
              frame 0, Default {
                n213 = local write "playlist"(i32[] [-1] ("playlist")) -> ()
              }
              frame 1 {
              }
            }
          }
          event Panel Close? {
            n214 = event-data() -> ()  [unwired: 1 in, 2 out]
            n215 = global write "musicplayer_glo.vi" "playlist sichtbar?"(FALSE ("playlist sichtbar?")) -> ()
            n216 = event-data("Discard?"=TRUE ("Verwerfen?")) -> ()  [unwired: 1 in, 1 out]
          }
        }
        n217 = case "sichtbarkeits-handler" shown="1" w136 {
          selector: w136 -> [w242 w250]
          tunnel: w135 -> [w243 w252]
          tunnel: [w241 w251] -> w134
          tunnel: w108 -> [w240 w249]
          frame 0, Default {
            n218 = case shown="False" w243 {
              tunnel: w242 -> [w245 w248]
              tunnel: [w244 w248] -> w241
              tunnel: w240 -> [w247 _]
              frame False {
                n219 = property class="VI"(reference=w247, "FP.State"=T3."Hidden" ("Frontpanel-Fenster:Status")) -> ()  [unwired: 1 in, 2 out]
                n220 = Increment(x=w245) -> (x+1=w244:i32)
              }
              frame True {
              }
            }
          }
          frame 1 {
            n221 = case shown="False" w252 {
              tunnel: [w253 0] -> w251
              tunnel: w250 -> [w253 _]
              tunnel: w249 -> [_ w254]
              frame False {
              }
              frame True {
                n222 = property class="VI"(reference=w254, "FP.State"=T3."Standard" ("Frontpanel-Fenster:Status")) -> ()  [unwired: 1 in, 2 out]
              }
            }
          }
        }
        n223 = case shown="True" w120 {
          tunnel: w118 -> [w181 _]
          tunnel: [w180 _] -> w119
          frame False {
            n224 = case shown="1" w181 {
              selector: w181 -> [w182 w187]
              tunnel: [w183 w187] -> w180
              frame 0, Default {
                n225 = Increment(x=w182) -> (x+1=w183:i32)
                n226 = control-ref of="Dieses VI"() -> (w186:refnum<vi>)
                n227 = property class="VI"(reference=w186, "FP.Behavior"=T5."Default" ("Frontpanel-Fenster:Verhaltensweise"), "Front Panel.Minimizeable"=TRUE ("Frontpanel-Fenster:Minimierbar")) -> ()  [unwired: 1 in, 2 out]
              }
              frame 1 {
              }
            }
          }
          frame True {
            n228 = control-ref of="Dieses VI"() -> (w189:refnum<vi>)
            n229 = property class="VI"(reference=w189) -> ("FP.State"=w191:T3)  [unwired: 1 in, 2 out]
            n230 = Equal?(x=w191, y=T3."Hidden") -> (x = y?=w188:bool)
            n231 = case shown="False" w188 {
              tunnel: w189 -> [w192 _]
              frame False {
                n232 = property class="VI"(reference=w192, "FP.State"=T3."Standard" ("Frontpanel-Fenster:Status"), "FP:RunTransparently"=TRUE ("Frontpanel-Fenster:VI transparent ausführen"), "FP.Behavior"=T5."Floating/Auto-Hide" ("Frontpanel-Fenster:Verhaltensweise"), "Front Panel.Minimizeable"=FALSE ("Frontpanel-Fenster:Minimierbar")) -> ()  [unwired: 1 in, 2 out]
              }
              frame True {
              }
            }
          }
        }
        n233 = case "abspielendezeile-handler" shown="True" w128 {
          tunnel: w127 -> [w220 w222]
          tunnel: [w220 w221] -> w126
          frame False {
          }
          frame True {
            n234 = stacked-sequence {
              tunnel: w222 -> [_ w225]
              tunnel: [_ w224] -> w221
              frame #0 {
                n235 = global write "musicplayer_glo.vi" "new-line-event-main"(FALSE ("new-line-event-main")) -> ()
              }
              frame #1 {
                w232 = u32 16382208 ("Farbfeld 2")
                n236 = property on="playlist" class="Listenfeld (strikt)"() -> ("Number of Rows"=w230:u32)  [unwired: 2 in, 2 out]
                n237 = global read "musicplayer_glo.vi" "new-line-event-main-line"() -> (w224:dbl)
                n238 = property on="playlist" class="Listenfeld (strikt)"("Active Row"=w225) -> ("CellBG"=w236:u32)  [unwired: 2 in, 2 out]
                n239 = Divide(x=w230, y=u32 2) -> (x/y=w226:dbl)
                n240 = global read "musicplayer_glo.vi" "follow-playing-titel?"() -> (w227:bool)
                n241 = Subtract(x=w224, y=w226) -> (x-y=w228:dbl)
                n242 = Not Equal?(x=w224, y=w225) -> (x != y?=w231:bool)
                n243 = Equal?(x=w236, y=w232) -> (x = y?=w235:bool)
                n244 = property on="playlist" class="Listenfeld (strikt)"("Active Row"=w224, "CellBG"=w232, "CellFontBold"=TRUE ("Aktive Zeile:Schriftart der Zelle:Fett")) -> ()  [unwired: 2 in, 2 out]
                n245 = case shown="True" w227 {
                  tunnel: w228 -> [_ w237]
                  frame False {
                  }
                  frame True {
                    n246 = property on="playlist" class="Listenfeld (strikt)"("Top Row"=w237) -> ()  [unwired: 2 in, 2 out]
                  }
                }
                n247 = And(x=w231, y=w235) -> (x .and. y?=w233:bool)
                n248 = case shown="True" w233 {
                  tunnel: w225 -> [_ w239]
                  frame False {
                  }
                  frame True {
                    n249 = property on="playlist" class="Listenfeld (strikt)"("Active Row"=w239, "CellBG"=u32 65280 ("Farbfeld 2")) -> ()  [unwired: 2 in, 2 out]
                  }
                }
              }
            }
          }
        }
        n250 = Or(x=w121, y=w110) -> (x .or. y?=w111:bool)
        n251 = case shown="False" w111 {
          frame False {
          }
          frame True {
            n252 = global read "musicplayer_glo.vi" "random?"() -> (w197:bool)
            n253 = case shown="True" w197 {
              frame False {
              }
              frame True {
                n254 = call "write_random_data.vi"() -> ()  [unwired: 12 in]
              }
            }
          }
        }
        n255 = global read "musicplayer_glo.vi" "exit?"() -> (w122:bool)
      }
    }
    frame #4 {
      n256 = flat-sequence {
        tunnel: w420 -> [w422]
        frame #0 {
          n257 = local read "win msg queue"() -> (w421:T1)
          n258 = call <userlib>:"Destroy Windows Message Queue.vi"("win msg queue"=w421) -> ()  [unwired: 1 in, 1 out]
        }
        frame #1 {
          n259 = invoke class="VI" method="FP.Schließen"(reference=w422) -> ()  [unwired: 2 in, 3 out]
        }
      }
    }
  }
